vi "ALTS-2015 Read INI file.vi"(8 "error in (no error)":errorcluster) -> (0 "error out":errorcluster)   [LabVIEW 2013]
doc: "Copyright © 2005, Soliton Technologies.\nAll rights reserved."
uses:
  Controls/ALTS-2015 LV2GBL Options.ctl
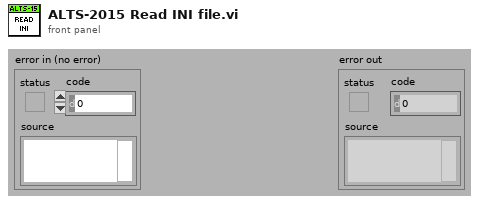
[diagram p1: front panel]
types:
  T1 = typedef "ALTS-2015 LV2GBL Options.ctl" = enum16{"Read all", "Write all"}
  T2 = typedef "ALTS-2015 INI Configuration Cluster.ctl" = cluster{"Application":cluster{"Rerun Count":i32, "Workorder No":string}, "Station Details":cluster{"Sensor Name 1":string, "Sensor Name 2":string, "Sensor Name 3":string, "Sensor Name 4":string, "Station1 Enable":bool, "Station2 Enable":bool, "Station3 Enable":bool, "Station4 Enable":bool}, "Database":cluster{"Database Connection Link":path, "Result Procedure":string, "User":string, "Password":string, "Prompt":bool, "Station 1 LT Result DB DSN Path":path, "Station 2 LT Result DB DSN Path":path, "Station 3 LT Result DB DSN Path":path, "Station 4 LT Result DB DSN Path":path, "AirLeakTestResult Procedure":string, "Serial Details Procedure":string}, "Simulation":cluster{"Simulate DAQ Hardware":bool, "Simulate Result DB Write":bool, "Simulate Scanner":bool, "Simulate OPC":bool, "Simulate Serial Details DB":bool, "Simulate Result DB":bool, "Simulate Scanner DB Path":path, "Simulate Serial Details DB Path":path, "Simulate Result DB Path":path}, "Barcode Scanner1":cluster{"Scanner IP":string, "Scanner Port":u16, "#Bytes to Read":i32}, "Barcode Scanner2":cluster{"Enabled?":bool, "Scanner IP":string, "Scanner Port":u16, "#Bytes to Read":i32}}
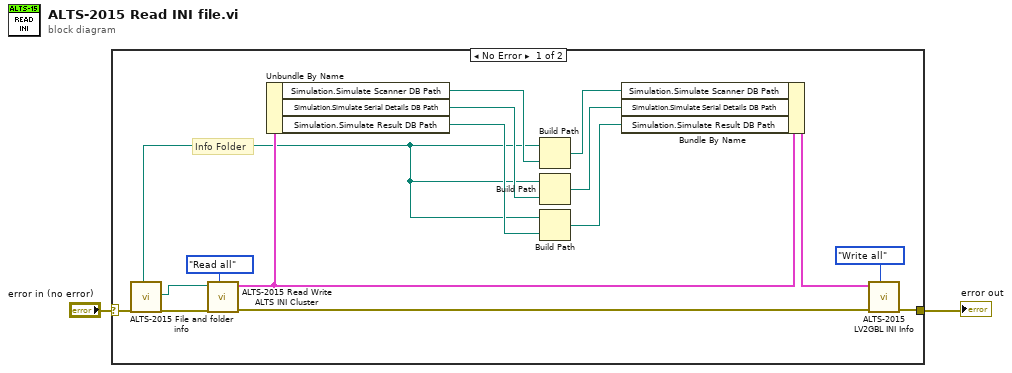
[diagram p0: block diagram]
diagram:
  n1 = case shown="No Error" "error in (no error)" {
    selector: "error in (no error)" -> [w14 w19]
    tunnel: [w13 w19] -> w1
    frame No Error {
      # "Info Folder"
      n2 = call "ALTS-2015 File and folder info.vi"("error in (no error)"=w14) -> ("Info Folder"=w3:path, "INI file path"=w11:path, "error out"=w15:errorcluster)  [unwired: 9 in, 7 out]
      n3 = call "ALTS-2015 Read Write ALTS INI Cluster.vi"("Options"=ALTS-2015_LV2GBL_Options."Read all", "error in (no error)"=w15, "INI File Path"=w11) -> ("error out"=w12:errorcluster, "Configuration Cluster Out"=w7:T2)  [unwired: 7 in]
      n4 = Unbundle By Name(w7) -> ("Simulation.Simulate Scanner DB Path"=w18:path, "Simulation.Simulate Serial Details DB Path"=w17:path, "Simulation.Simulate Result DB Path"=w16:path)
      n5 = Build Path(base path=w3, name or relative path=w18) -> (appended path=w5:path)
      n6 = Build Path(base path=w3, name or relative path=w17) -> (appended path=w6:path)
      n7 = Build Path(base path=w3, name or relative path=w16) -> (appended path=w4:path)
      n8 = Bundle By Name(cluster=w7, "Simulation.Simulate Scanner DB Path"=w5, "Simulation.Simulate Serial Details DB Path"=w6, "Simulation.Simulate Result DB Path"=w4) -> (w8:T2)
      n9 = call "ALTS-2015 LV2GBL INI Info.vi"("Options"=ALTS-2015_LV2GBL_Options."Write all", "error in"=w12, "Configuration Cluster"=w8) -> ("error out"=w13:errorcluster)  [unwired: 7 in, 1 out]
    }
    frame Error {
    }
  }
  "error out" <- w1
